vi "题2.vi"() -> ()   [LabVIEW 2017]
panel:
  in  "数字数据":digitaldata
  out "数字波形图":digitaldata(graph)
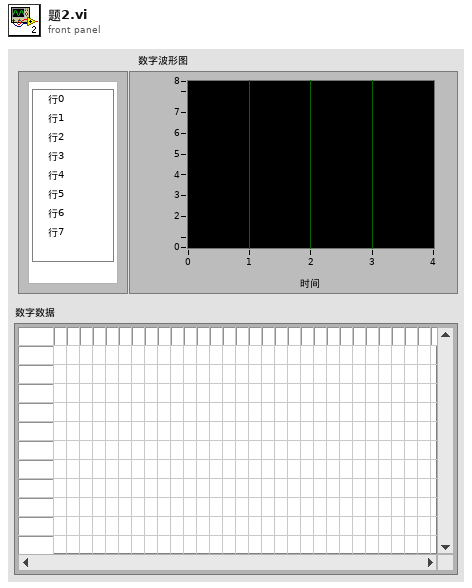
[diagram p1: front panel]
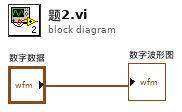
[diagram p0: block diagram]
diagram:
  "数字波形图" <- "数字数据"
